vi "setWriteFIFO.vi"(10 "WriteFIFO":refnum<class "IWriteFIFO.lvclass">, 11 "Modbus in":refnum<class "Modbus.lvclass">) -> (3 "Modbus out":refnum<class "Modbus.lvclass">)   [LabVIEW 2015, in "RTModbus.lvlib" / "Modbus.lvclass"]
uses:
  Modbus.lvclass
  Common_RT_FPGA/IWriteFIFO/IWriteFIFO.lvclass
  Modbus.lvclass/Modbus.ctl
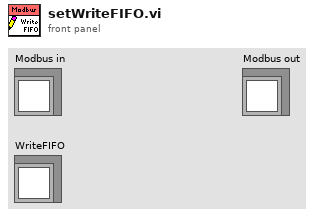
[diagram p1: front panel]
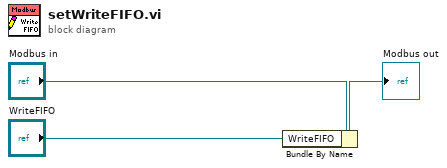
[diagram p0: block diagram]
diagram:
  n1 = Bundle By Name(cluster="Modbus in", "WriteFIFO"="WriteFIFO") -> (→"Modbus out":refnum<class "Modbus.lvclass">)
